vi "PTScanner.ProcCases.vi"(0 "i ref in":refnum<vi>, 1 "selector":string, 2 "Data":T3, 3 "call cluster":T1={"Object"="", "Selector"="", "CallType"=enum."synchronous", "Async Object"="", "Async Selector"="", "Data Descriptor"="", "Data"=[], "Error #"=0, "Expire"=0}, 5 "error in (no error)":errorcluster) -> (14 "i ref out":refnum<vi>, 17 "answer cluster":T1={"Object"="", "Selector"="", "CallType"=enum."synchronous", "Async Object"="", "Async Selector"="", "Data Descriptor"="", "Data"=[], "Error #"=0, "Expire"=0}, 19 "error out":errorcluster)   [LabVIEW 2014, in "PTScanner.lvlib"]
uses:
  PTScanner.lvlib
  CS_Core/CSSystem/CoreDefs/CoreDefs.rawDataType.ctl
  CS_Core/CSSystem/CoreDefs/CoreDefs.call_type.ctl
  CS_Core/BaseProcess/BaseProcess.descriptor string definition.ctl
  CS_Core/CSSystem/CoreLib/CoreLib.string 2 byte array.vi
  CS_Core/CSSystem/CoreLib/CoreLib.byte array 2 string.vi
  <vilib>/Utility/xml.llb/Write to XML File(string).vi
  <vilib>/Utility/xml.llb/Read From XML File(string).vi
  CS_Core/CSSystem/CoreLib/CoreLib.short 2 byte array.vi
  CS_Core/BaseProcess/BaseProcess.lvlib
  CS_Core/CSSystem/CoreLib/CoreLib.lvlib
  CS_Core/CAEObj/CAEObj.lvlib
  CSlibraries-extern/DimLVEvent/LVDimInterface/LVDimInterface.lvlib
  CS_Core/BaseSM/BaseSM.lvlib
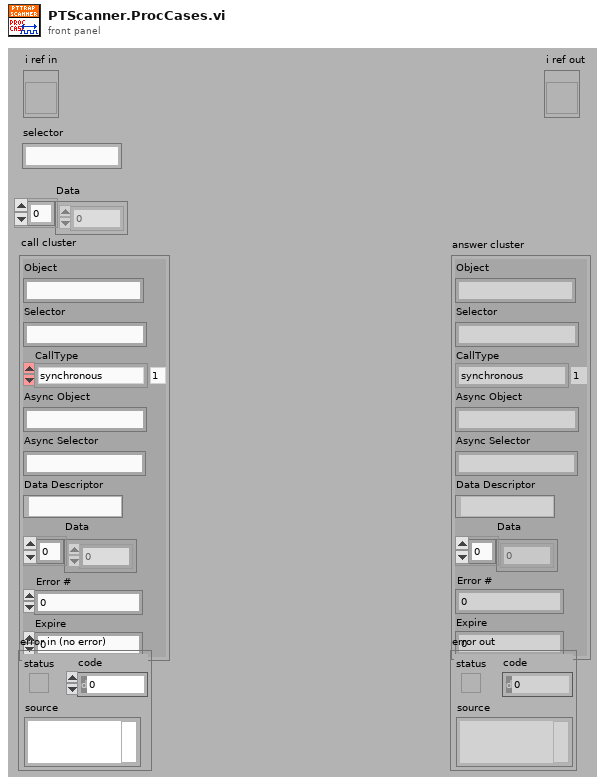
[diagram p1: front panel]
types:
  T1 = typedef "CoreDefs.call_type.ctl" = cluster{"Object":string, "Selector":string, "CallType":enum16{"simple", "synchronous", "asynchronous"}, "Async Object":string, "Async Selector":string, "Data Descriptor":T2, "Data":T3, "Error #":i32, "Expire":u32}
  T2 = typedef "BaseProcess.lvlib/BaseProcess.descriptor string definition.ctl" = string
  T3 = typedef "CoreDefs.rawDataType.ctl" = i8[]
  T4 = typedef "PTScanner.lvlib/PTScanner.i attribute.ctl" = cluster{"Object cmds":T5[], "Steps":cluster{"Finished":bool, "cmd setup":T6[]}[], "curStep":i32, "DIM IDs":cluster{"AllFinished":i32, "Finished":i32, "curStep":i32, "nofSteps":i32, "NomValues":i32[], "1D-Min":i32, "1D-Max":i32, "Dimensions":i32, "MaxDimensions":i32, "ScanedDeviceNames":i32[]}, "All Finished":bool, "DIMs in use":string[], "Running":bool, "Scan Delay":u32, "loop":bool, "Paused":bool, "Formed":bool}
  T5 = typedef "PTScanner.lvlib/PTScanner.obj parameters.ctl" = cluster{"object":string, "DIM address":string, "method":string, "data descriptor":string, "method parameters":cluster{"Name":string, "Descr":string, "Value":string, "Value?":bool}[], "Call Mode":enum16{"Simple DIM", "Synchronous"}, "actValue":dbl, "Centroid":dbl, "Minus Delta":dbl, "Plus Delta":dbl, "increment":dbl, "DIM Status":cluster{"no link":bool, "quality":i32, "Time Stamp":timestamp}, "range":dbl, "DIMChannelIndex":i32}
  T6 = typedef "PTScanner.lvlib/PTScanner.step obj parameters.ctl" = cluster{"obj index":i32, "nomValue":dbl, "fulfilled":bool}
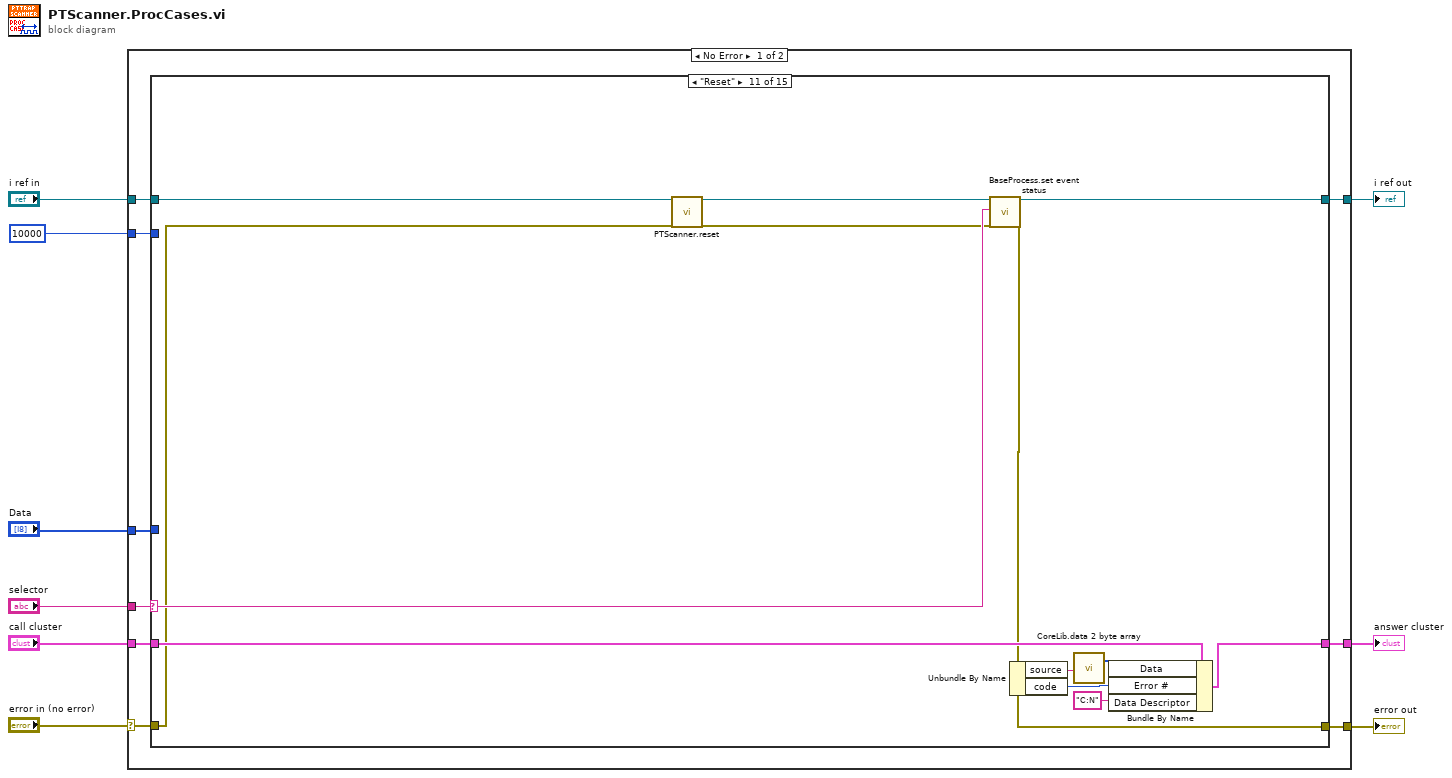
[diagram p0: block diagram]
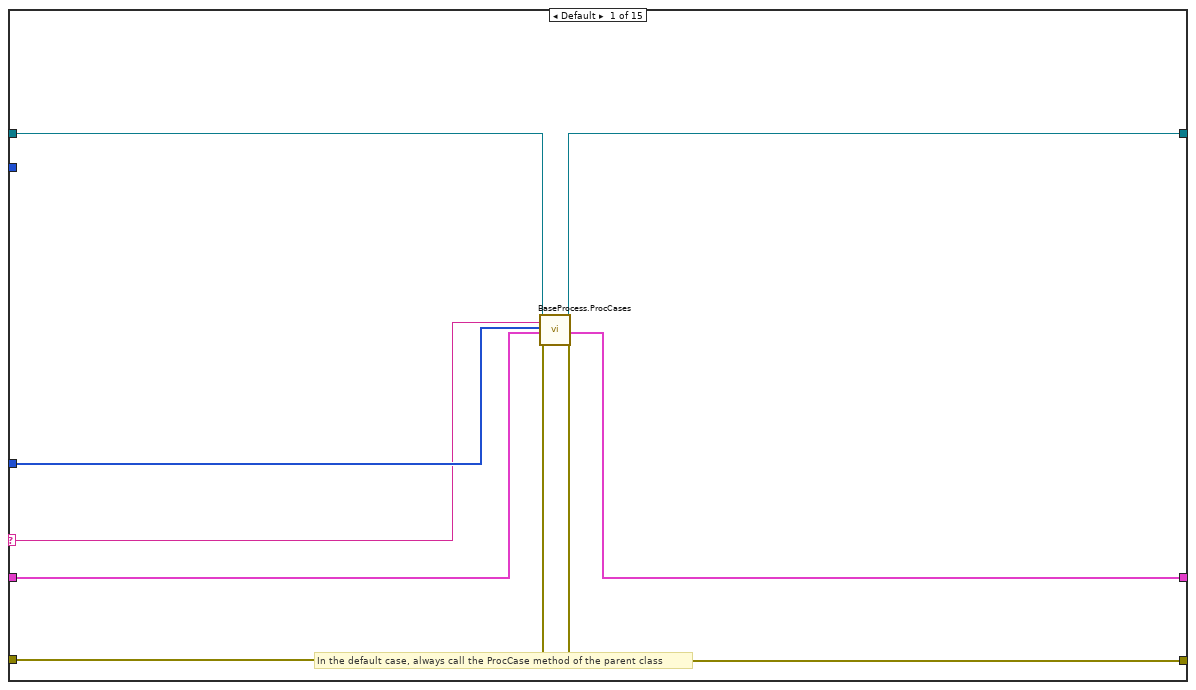
[diagram p2: hidden frame]
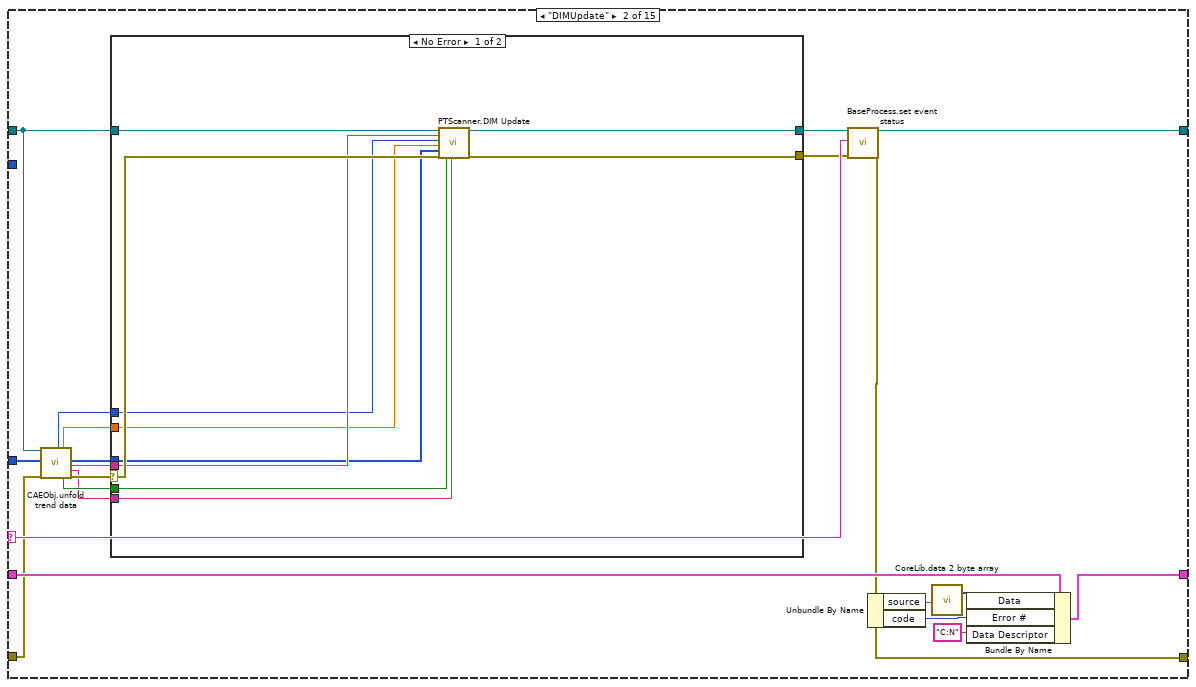
[diagram p3: hidden frame]
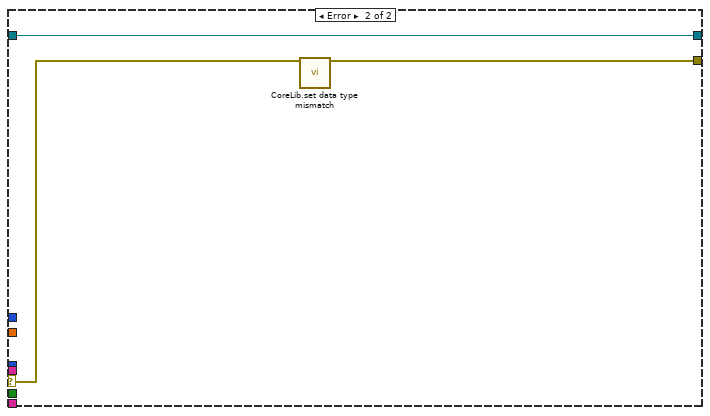
[diagram p4: hidden frame]
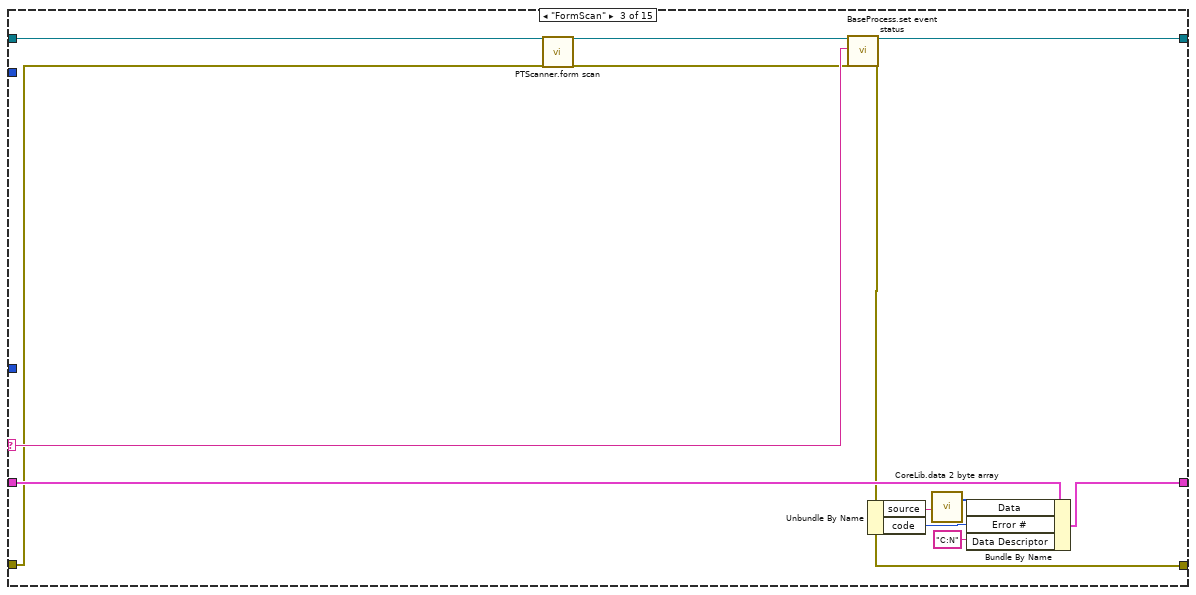
[diagram p5: hidden frame]
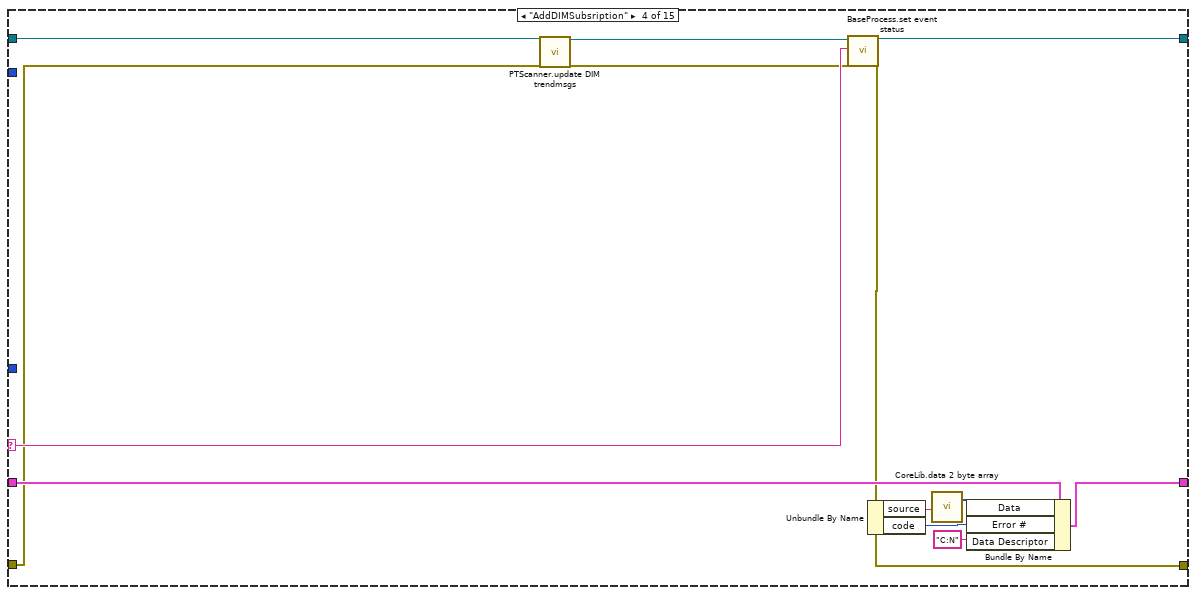
[diagram p6: hidden frame]
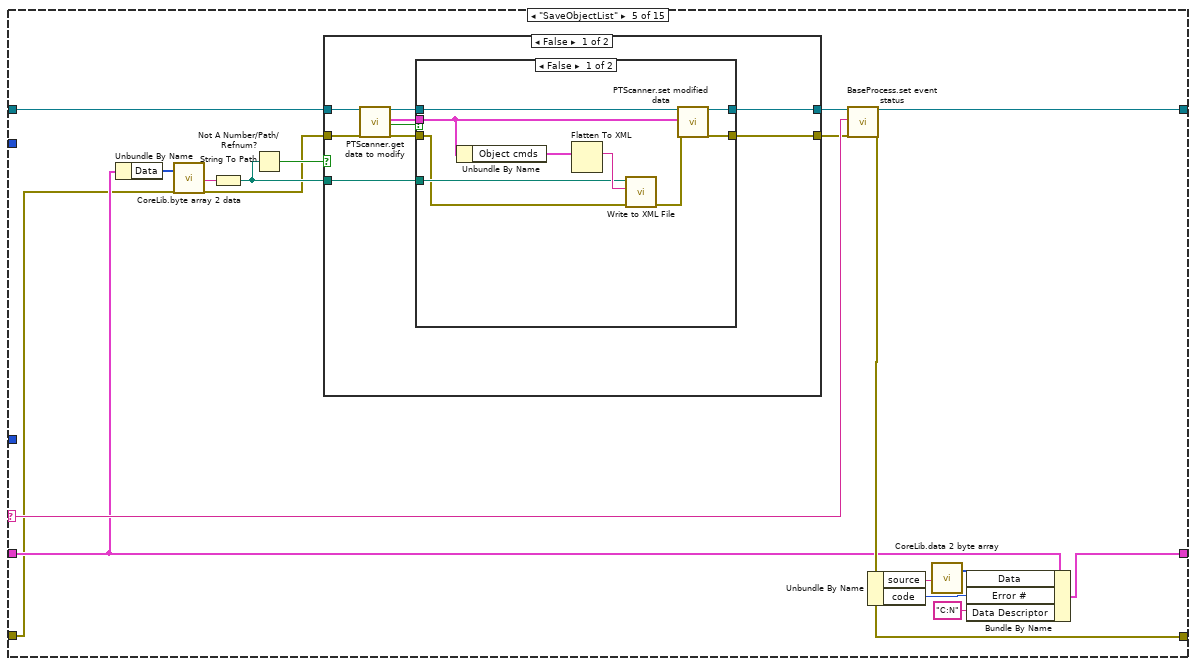
[diagram p7: hidden frame]
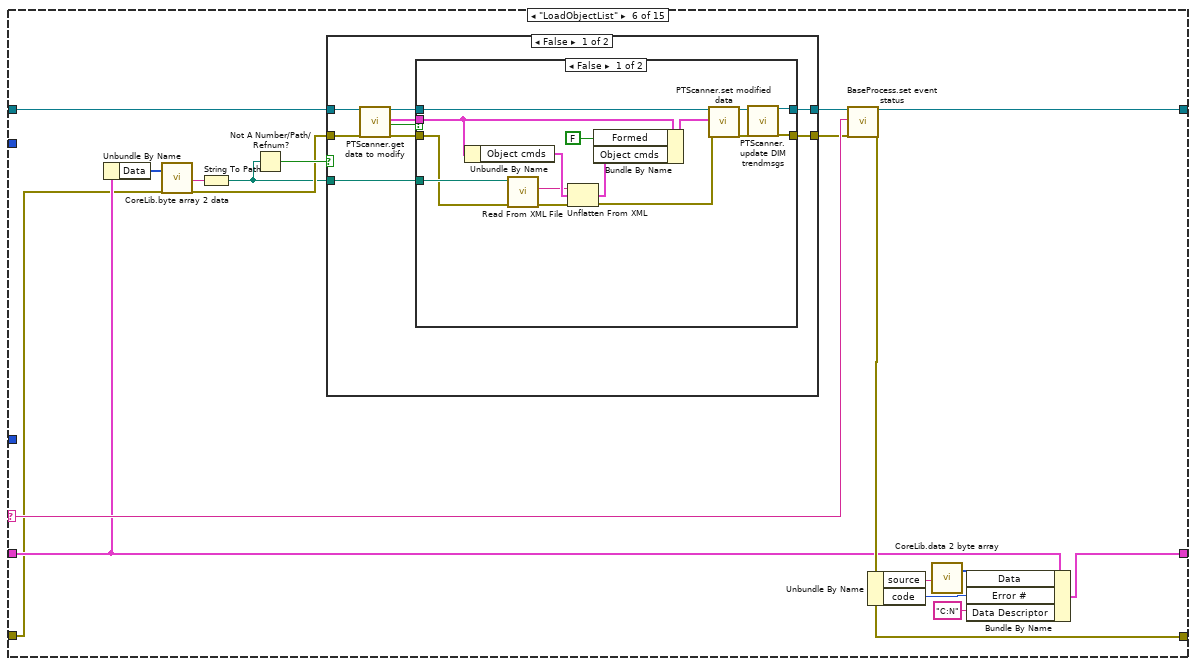
[diagram p10: hidden frame]
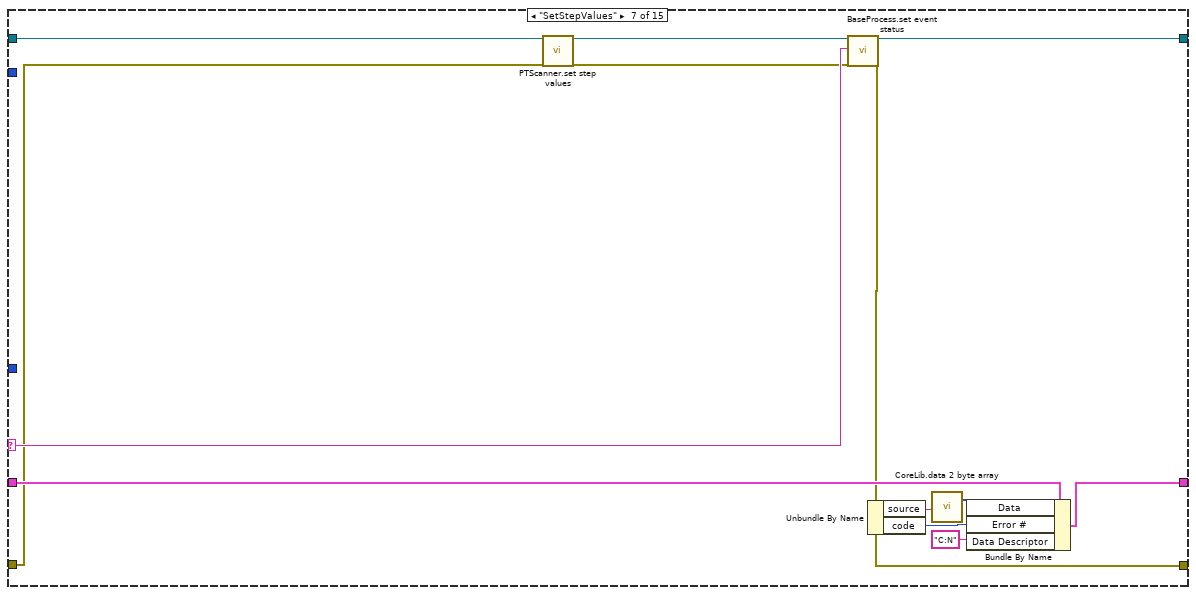
[diagram p13: hidden frame]
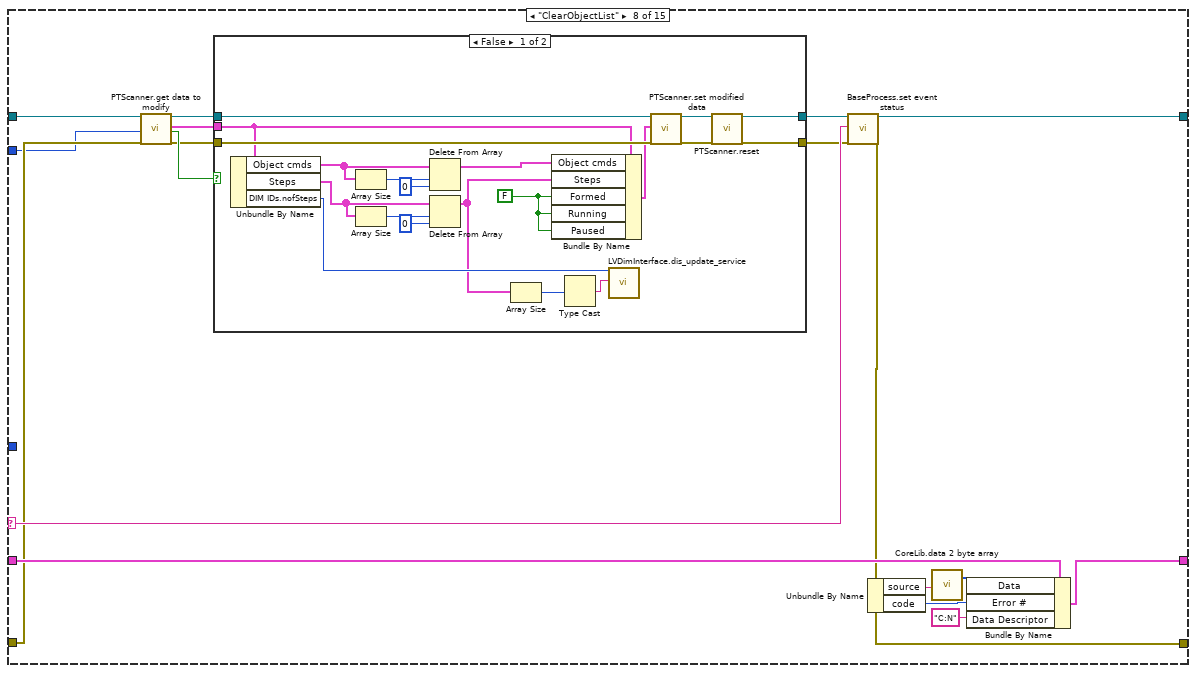
[diagram p14: hidden frame]
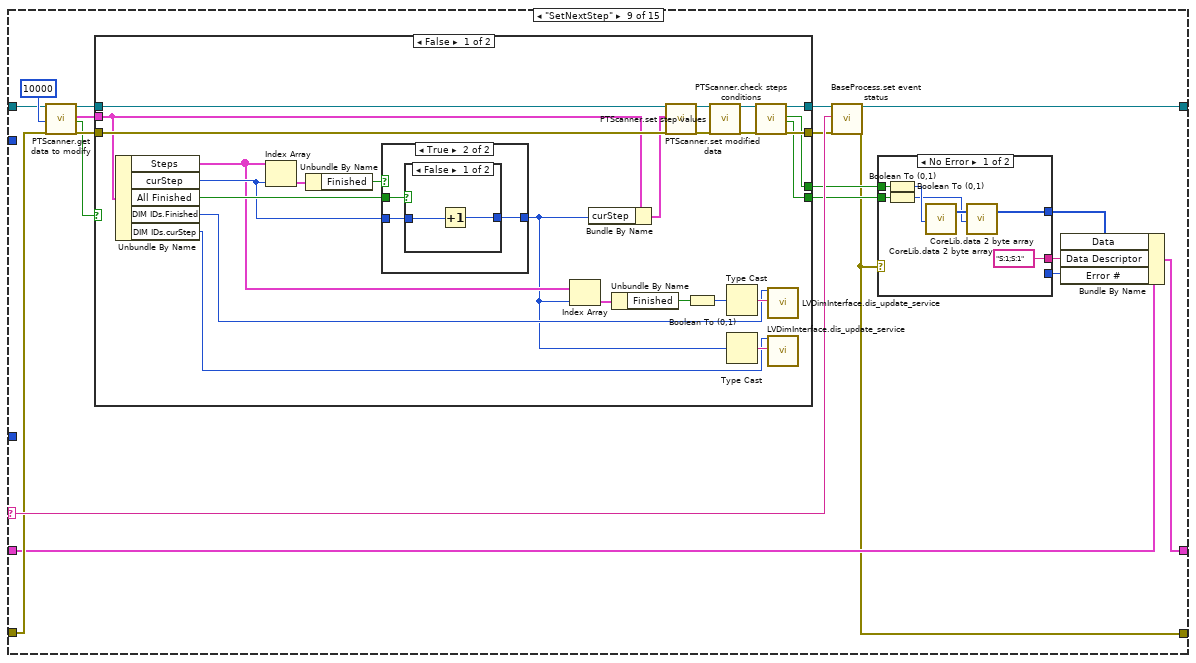
[diagram p16: hidden frame]
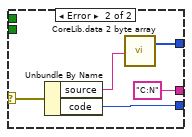
[diagram p17: hidden frame]
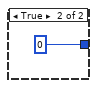
[diagram p19: hidden frame]
diagram:
  n1 = case shown="No Error" "error in (no error)" {
    selector: "error in (no error)" -> [w10 w504]
    tunnel: "selector" -> [w18 _]
    tunnel: [w17 w505] -> w8
    tunnel: "Data" -> [w16 _]
    tunnel: "call cluster" -> [w15 w505]
    tunnel: "i ref in" -> [w14 w506]
    tunnel: [w13 w506] -> w4
    tunnel: [w12 w504] -> w3
    tunnel: 10000 -> [w11 _]
    frame No Error {
      n2 = case shown="\"Reset\"" w18 {
        selector: w18 -> [w20 w39 w67 w80 w99 w139 w179 w197 w244 w306 w365 w378 w396 w451 w478]
        tunnel: w16 -> [w21 w38 _ _ _ _ _ _ _ _ _ _ _ _ _]
        tunnel: w14 -> [w19 w31 w65 w76 w88 w131 w177 w195 w235 w302 w362 w375 w392 w447 w474]
        tunnel: [w26 w41 w66 w79 w98 w138 w178 w196 w243 w305 w364 w377 w395 w450 w477] -> w13
        tunnel: w15 -> [w22 w43 w69 w82 w91 w134 w181 w199 w227 w307 w367 w380 w398 w453 w480]
        tunnel: [w23 w42 w70 w83 w101 w141 w182 w200 w228 w308 w368 w381 w399 w454 w481] -> w17
        tunnel: w10 -> [w25 w36 w64 w75 w90 w130 w174 w194 w234 w300 w361 w372 w390 w445 w472]
        tunnel: [w24 w40 w68 w81 w100 w140 w180 w198 w226 w295 w366 w379 w397 w452 w479] -> w12
        tunnel: w11 -> [_ _ _ _ _ _ _ w193 _ _ _ _ _ _ _]
        frame Default {
          # "In the default case, always call the ProcCase method of the parent class"
          n3 = call "BaseProcess.ProcCases.vi"("i ref in"=w19, "selector"=w20, "Data"=w21, "call cluster"=w22, "error in (no error)"=w25) -> ("i ref out"=w26:refnum<vi>, "answer cluster"=w23:T1, "error out"=w24:errorcluster)  [unwired: 12 in]
        }
        frame "DIMUpdate" {
          n4 = call "CAEObj.unfold trend data.vi"("i ref in"=w31, "raw trend data"=w38, "error in (no error)"=w36) -> ("quality"=w33:i32, "timeStamp"=w34:dbl, "no link"=w29:bool, "data"=w35:i8[], "serviceName"=w28:string, "typeDescriptor"=w27:string, "error out"=w37:errorcluster)  [unwired: 8 in, 2 out]
          n5 = case shown="No Error" w37 {
            selector: w37 -> [w54 w59]
            tunnel: w35 -> [w51 _]
            tunnel: w34 -> [w49 _]
            tunnel: w33 -> [w50 _]
            tunnel: [w55 w60] -> w32
            tunnel: w31 -> [w57 w58]
            tunnel: [w56 w58] -> w30
            tunnel: w29 -> [w53 _]
            tunnel: w28 -> [w52 _]
            tunnel: w27 -> [w48 _]
            frame No Error {
              n6 = call "PTScanner.DIM Update.vi"("i ref in"=w57, "serviceName"=w52, "quality"=w50, "Time Stamp"=w49, "data"=w51, "error in (no error)"=w54, "no link"=w53, "typeDescriptor"=w48) -> ("i ref out"=w56:refnum<vi>, "error out"=w55:errorcluster)  [unwired: 10 in]
            }
            frame Error {
              n7 = call "CoreLib.set data type mismatch.vi"("error in (no error)"=w59) -> ("error out"=w60:errorcluster)  [unwired: 18 in]
            }
          }
          n8 = call "BaseProcess.set event status.vi"("i ref in"=w30, "EventStatus"=w39, "error in (no error)"=w32) -> ("i ref out"=w41:refnum<vi>, "error out"=w40:errorcluster)  [unwired: 14 in, 1 out]
          n9 = Unbundle By Name(w40) -> ("source"=w44:string, "code"=w47:i32)
          n10 = call-poly "CoreLib.data 2 byte array.vi"("string"=w44) -> ("byteArray out"=w46:T3)  [unwired: 18 in]
          n11 = Bundle By Name(cluster=w43, "Data"=w46, "Error #"=w47, "Data Descriptor"="C:N") -> (w42:T1)
        }
        frame "FormScan" {
          n12 = call "PTScanner.form scan.vi"("i ref in"=w65, "error in (no error)"=w64) -> ("i ref out"=w63:refnum<vi>, "error out"=w62:errorcluster)  [unwired: 16 in]
          n13 = call "BaseProcess.set event status.vi"("i ref in"=w63, "EventStatus"=w67, "error in (no error)"=w62) -> ("i ref out"=w66:refnum<vi>, "error out"=w68:errorcluster)  [unwired: 14 in, 1 out]
          n14 = Unbundle By Name(w68) -> ("source"=w61:string, "code"=w73:i32)
          n15 = call-poly "CoreLib.data 2 byte array.vi"("string"=w61) -> ("byteArray out"=w72:T3)  [unwired: 18 in]
          n16 = Bundle By Name(cluster=w69, "Data"=w72, "Error #"=w73, "Data Descriptor"="C:N") -> (w70:T1)
        }
        frame "AddDIMSubsription" {
          n17 = call "PTScanner.update DIM trendmsgs.vi"("i ref in"=w76, "error in"=w75) -> ("i ref out"=w78:refnum<vi>, "error out"=w77:errorcluster)  [unwired: 16 in]
          n18 = call "BaseProcess.set event status.vi"("i ref in"=w78, "EventStatus"=w80, "error in (no error)"=w77) -> ("i ref out"=w79:refnum<vi>, "error out"=w81:errorcluster)  [unwired: 14 in, 1 out]
          n19 = Unbundle By Name(w81) -> ("source"=w74:string, "code"=w86:i32)
          n20 = call-poly "CoreLib.data 2 byte array.vi"("string"=w74) -> ("byteArray out"=w85:T3)  [unwired: 18 in]
          n21 = Bundle By Name(cluster=w82, "Data"=w85, "Error #"=w86, "Data Descriptor"="C:N") -> (w83:T1)
        }
        frame "SaveObjectList" {
          n22 = Unbundle By Name(w91) -> ("Data"=w95:T3)
          n23 = call-poly "CoreLib.byte array 2 data.vi"("byteArray"=w95, "error in (no error)"=w90) -> ("string"=w94:string, "error out"=w89:errorcluster)  [unwired: 15 in, 1 out]
          n24 = String To Path(string=w94) -> (path=w93:path)
          n25 = Not A Number/Path/Refnum?(number/path/refnum=w93) -> (NaN/Path/Refnum?=w92:bool)
          n26 = case shown="False" w92 {
            tunnel: w89 -> [w110 w125]
            tunnel: w88 -> [w113 w126]
            tunnel: w93 -> [w109 _]
            tunnel: [w107 w126] -> w97
            tunnel: [w105 w125] -> w96
            frame False {
              n27 = call "PTScanner.get data to modify.vi"("i ref in"=w113, "error in (no error)"=w110) -> ("i ref out"=w108:refnum<vi>, "i attribute"=w111:T4, "timed out"=w112:bool, "error out"=w106:errorcluster)  [unwired: 14 in]
              n28 = case shown="False" w112 {
                tunnel: w111 -> [w117 _]
                tunnel: w109 -> [w120 _]
                tunnel: [w119 w124] -> w107
                tunnel: w108 -> [w118 w124]
                tunnel: w106 -> [w116 w123]
                tunnel: [w114 w123] -> w105
                frame False {
                  n29 = Unbundle By Name(w117) -> ("Object cmds"=w122:T5[])
                  n30 = Flatten To XML(anything=w122) -> (xml string=w121:string)
                  n31 = call-poly <vilib>:"Write to XML File.vi"("error in (no error)"=w116, "XML Input"=w121, "XML File Path"=w120) -> ("error out"=w115:errorcluster)  [unwired: 6 in, 2 out]
                  n32 = call "PTScanner.set modified data.vi"("i ref in"=w118, "CLASS.i attribute"=w117, "error in (no error)"=w115) -> ("i ref out"=w119:refnum<vi>, "error out"=w114:errorcluster)  [unwired: 15 in]
                }
                frame True {
                }
              }
            }
            frame True {
            }
          }
          n33 = call "BaseProcess.set event status.vi"("i ref in"=w97, "EventStatus"=w99, "error in (no error)"=w96) -> ("i ref out"=w98:refnum<vi>, "error out"=w100:errorcluster)  [unwired: 14 in, 1 out]
          n34 = Unbundle By Name(w100) -> ("source"=w87:string, "code"=w104:i32)
          n35 = call-poly "CoreLib.data 2 byte array.vi"("string"=w87) -> ("byteArray out"=w103:T3)  [unwired: 18 in]
          n36 = Bundle By Name(cluster=w91, "Data"=w103, "Error #"=w104, "Data Descriptor"="C:N") -> (w101:T1)
        }
        frame "LoadObjectList" {
          n37 = Unbundle By Name(w134) -> ("Data"=w135:T3)
          n38 = call-poly "CoreLib.byte array 2 data.vi"("byteArray"=w135, "error in (no error)"=w130) -> ("string"=w133:string, "error out"=w129:errorcluster)  [unwired: 15 in, 1 out]
          n39 = String To Path(string=w133) -> (path=w128:path)
          n40 = Not A Number/Path/Refnum?(number/path/refnum=w128) -> (NaN/Path/Refnum?=w132:bool)
          n41 = case shown="False" w132 {
            tunnel: w129 -> [w150 w171]
            tunnel: w131 -> [w153 w172]
            tunnel: [w148 w172] -> w137
            tunnel: [w146 w171] -> w136
            tunnel: w128 -> [w145 _]
            frame False {
              n42 = call "PTScanner.get data to modify.vi"("i ref in"=w153, "error in (no error)"=w150) -> ("i ref out"=w149:refnum<vi>, "i attribute"=w151:T4, "timed out"=w152:bool, "error out"=w147:errorcluster)  [unwired: 14 in]
              n43 = case shown="False" w152 {
                tunnel: w151 -> [w163 _]
                tunnel: w145 -> [w168 _]
                tunnel: [w156 w170] -> w148
                tunnel: w149 -> [w167 w170]
                tunnel: w147 -> [w166 w169]
                tunnel: [w155 w169] -> w146
                frame False {
                  n44 = Unbundle By Name(w163) -> ("Object cmds"=w161:T5[])
                  n45 = call-poly <vilib>:"Read From XML File.vi"("error in (no error)"=w166, "XML File Path"=w168) -> ("error out"=w165:errorcluster, "XML Elements"=w160:string)  [unwired: 7 in, 1 out]
                  n46 = Unflatten From XML(xml string=w160, type=w161, error in (no error)=w165) -> (value=w162:T5[], error out=w164:errorcluster)
                  n47 = Bundle By Name(cluster=w163, "Formed"=FALSE, "Object cmds"=w162) -> (w159:T4)
                  n48 = call "PTScanner.set modified data.vi"("i ref in"=w167, "CLASS.i attribute"=w159, "error in (no error)"=w164) -> ("i ref out"=w158:refnum<vi>, "error out"=w157:errorcluster)  [unwired: 15 in]
                  n49 = call "PTScanner.update DIM trendmsgs.vi"("i ref in"=w158, "error in"=w157) -> ("i ref out"=w156:refnum<vi>, "error out"=w155:errorcluster)  [unwired: 16 in]
                }
                frame True {
                }
              }
            }
            frame True {
            }
          }
          n50 = call "BaseProcess.set event status.vi"("i ref in"=w137, "EventStatus"=w139, "error in (no error)"=w136) -> ("i ref out"=w138:refnum<vi>, "error out"=w140:errorcluster)  [unwired: 14 in, 1 out]
          n51 = Unbundle By Name(w140) -> ("source"=w127:string, "code"=w144:i32)
          n52 = call-poly "CoreLib.data 2 byte array.vi"("string"=w127) -> ("byteArray out"=w143:T3)  [unwired: 18 in]
          n53 = Bundle By Name(cluster=w134, "Data"=w143, "Error #"=w144, "Data Descriptor"="C:N") -> (w141:T1)
        }
        frame "SetStepValues" {
          n54 = call "PTScanner.set step values.vi"("i ref in"=w177, "error in(no error)"=w174) -> ("i ref out"=w176:refnum<vi>, "error out"=w175:errorcluster)  [unwired: 16 in]
          n55 = call "BaseProcess.set event status.vi"("i ref in"=w176, "EventStatus"=w179, "error in (no error)"=w175) -> ("i ref out"=w178:refnum<vi>, "error out"=w180:errorcluster)  [unwired: 14 in, 1 out]
          n56 = Unbundle By Name(w180) -> ("source"=w173:string, "code"=w185:i32)
          n57 = call-poly "CoreLib.data 2 byte array.vi"("string"=w173) -> ("byteArray out"=w184:T3)  [unwired: 18 in]
          n58 = Bundle By Name(cluster=w181, "Data"=w184, "Error #"=w185, "Data Descriptor"="C:N") -> (w182:T1)
        }
        frame "ClearObjectList" {
          n59 = call "PTScanner.get data to modify.vi"("i ref in"=w195, "ms timeout (10000)"=w193, "error in (no error)"=w194) -> ("i ref out"=w191:refnum<vi>, "i attribute"=w187:T4, "timed out"=w192:bool, "error out"=w190:errorcluster)  [unwired: 13 in]
          n60 = case shown="False" w192 {
            tunnel: w191 -> [w223 w225]
            tunnel: w190 -> [w222 w224]
            tunnel: [w210 w224] -> w189
            tunnel: [w209 w225] -> w188
            tunnel: w187 -> [w217 _]
            frame False {
              w208 = FALSE
              n61 = Unbundle By Name(w217) -> ("Object cmds"=w220:T5[], "Steps"=w213:cluster{"Finished":bool, "cmd setup":T6[]}[], "DIM IDs.nofSteps"=w206:i32)
              n62 = Array Size(array=w220) -> (size(s)=w221:i32)
              n63 = Array Size(array=w213) -> (size(s)=w214:i32)
              n64 = Delete From Array(array=w220, length=w221, index=0) -> (array with subset deleted=w218:T5[])  [unwired: 1 out]
              n65 = Delete From Array(array=w213, length=w214, index=0) -> (array with subset deleted=w205:cluster{"Finished":bool, "cmd setup":T6[]}[])  [unwired: 1 out]
              n66 = Array Size(array=w205) -> (size(s)=w204:i32)
              n67 = Bundle By Name(cluster=w217, "Object cmds"=w218, "Steps"=w205, "Formed"=w208, "Running"=w208, "Paused"=w208) -> (w216:T4)
              n68 = Type Cast(x=w204) -> (*(type *) &x=w207:string)  [unwired: 1 in]
              n69 = call "LVDimInterface.dis_update_service.vi"("my_serviceID"=w206, "data"=w207) -> ()  [unwired: 15 in, 3 out]
              n70 = call "PTScanner.set modified data.vi"("i ref in"=w223, "CLASS.i attribute"=w216, "error in (no error)"=w222) -> ("i ref out"=w212:refnum<vi>, "error out"=w211:errorcluster)  [unwired: 15 in]
              n71 = call "PTScanner.reset.vi"("i ref in"=w212, "error in (no error)"=w211) -> ("i ref out"=w209:refnum<vi>, "error out"=w210:errorcluster)  [unwired: 16 in]
            }
            frame True {
            }
          }
          n72 = call "BaseProcess.set event status.vi"("i ref in"=w188, "EventStatus"=w197, "error in (no error)"=w189) -> ("i ref out"=w196:refnum<vi>, "error out"=w198:errorcluster)  [unwired: 14 in, 1 out]
          n73 = Unbundle By Name(w198) -> ("source"=w186:string, "code"=w203:i32)
          n74 = call-poly "CoreLib.data 2 byte array.vi"("string"=w186) -> ("byteArray out"=w202:T3)  [unwired: 18 in]
          n75 = Bundle By Name(cluster=w199, "Data"=w202, "Error #"=w203, "Data Descriptor"="C:N") -> (w200:T1)
        }
        frame "SetNextStep" {
          n76 = call "PTScanner.get data to modify.vi"("i ref in"=w235, "ms timeout (10000)"=10000, "error in (no error)"=w234) -> ("i ref out"=w240:refnum<vi>, "i attribute"=w236:T4, "timed out"=w237:bool, "error out"=w239:errorcluster)  [unwired: 13 in]
          n77 = case shown="False" w237 {
            tunnel: w240 -> [w281 w290]
            tunnel: [w262 w290] -> w242
            tunnel: [w263 w289] -> w241
            tunnel: w239 -> [w280 w289]
            tunnel: w236 -> [w278 _]
            tunnel: [w261 _] -> w229
            tunnel: [w260 _] -> w230
            frame False {
              n78 = Unbundle By Name(w278) -> ("Steps"=w270:cluster{"Finished":bool, "cmd setup":T6[]}[], "curStep"=w274:i32, "All Finished"=w276:bool, "DIM IDs.Finished"=w267:i32, "DIM IDs.curStep"=w258:i32)
              n79 = Index Array(array=w270, index=w274) -> (element=w275:cluster{"Finished":bool, "cmd setup":T6[]})
              n80 = Unbundle By Name(w275) -> ("Finished"=w273:bool)
              n81 = case shown="True" w273 {
                tunnel: w276 -> [_ w285]
                tunnel: [w282 w284] -> w257
                tunnel: w274 -> [w282 w283]
                frame False {
                }
                frame True {
                  n82 = case shown="False" w285 {
                    tunnel: [w287 0] -> w284
                    tunnel: w283 -> [w286 _]
                    frame False {
                      n83 = Increment(x=w286) -> (x+1=w287:i32)
                    }
                    frame True {
                    }
                  }
                }
              }
              n84 = Index Array(array=w270, index=w257) -> (element=w269:cluster{"Finished":bool, "cmd setup":T6[]})
              n85 = Bundle By Name(cluster=w278, "curStep"=w257) -> (w277:T4)
              n86 = Unbundle By Name(w269) -> ("Finished"=w268:bool)
              n87 = call "PTScanner.set modified data.vi"("i ref in"=w281, "CLASS.i attribute"=w277, "error in (no error)"=w280) -> ("i ref out"=w266:refnum<vi>, "error out"=w279:errorcluster)  [unwired: 15 in]
              n88 = Boolean To (0,1)(Boolean=w268) -> (0, 1=w271:i16)
              n89 = call "PTScanner.set step values.vi"("i ref in"=w266, "error in(no error)"=w279) -> ("i ref out"=w265:refnum<vi>, "error out"=w264:errorcluster)  [unwired: 16 in]
              n90 = Type Cast(x=w271) -> (*(type *) &x=w272:string)  [unwired: 1 in]
              n91 = Type Cast(x=w257) -> (*(type *) &x=w259:string)  [unwired: 1 in]
              n92 = call "PTScanner.check steps conditions.vi"("i ref in"=w265, "error in (no error)"=w264) -> ("i ref out"=w262:refnum<vi>, "Finished"=w261:bool, "All Finished"=w260:bool, "error out"=w263:errorcluster)  [unwired: 14 in]
              n93 = call "LVDimInterface.dis_update_service.vi"("my_serviceID"=w267, "data"=w272) -> ()  [unwired: 15 in, 3 out]
              n94 = call "LVDimInterface.dis_update_service.vi"("my_serviceID"=w258, "data"=w259) -> ()  [unwired: 15 in, 3 out]
            }
            frame True {
            }
          }
          n95 = call "BaseProcess.set event status.vi"("i ref in"=w242, "EventStatus"=w244, "error in (no error)"=w241) -> ("i ref out"=w243:refnum<vi>, "error out"=w226:errorcluster)  [unwired: 14 in, 1 out]
          n96 = case shown="No Error" w226 {
            selector: w226 -> [_ w253]
            tunnel: [_ w256] -> w231
            tunnel: [w245 w255] -> w233
            tunnel: w229 -> [w250 _]
            tunnel: w230 -> [w249 _]
            tunnel: ["S:1;S:1" ("Data Descriptor") "C:N" ("Data Descriptor")] -> w232
            frame No Error {
              n97 = Boolean To (0,1)(Boolean=w250) -> (0, 1=w248:i16)
              n98 = Boolean To (0,1)(Boolean=w249) -> (0, 1=w247:i16)
              n99 = call-poly "CoreLib.data 2 byte array.vi"("i16"=w248) -> ("byteArray out"=w251:T3)  [unwired: 18 in]
              n100 = call-poly "CoreLib.data 2 byte array.vi"("byteArray"=w251, "i16"=w247) -> ("byteArray out"=w245:T3)  [unwired: 17 in]
            }
            frame Error {
              n101 = Unbundle By Name(w253) -> ("source"=w254:string, "code"=w256:i32)
              n102 = call-poly "CoreLib.data 2 byte array.vi"("string"=w254) -> ("byteArray out"=w255:T3)  [unwired: 18 in]
            }
          }
          n103 = Bundle By Name(cluster=w227, "Data"=w233, "Data Descriptor"=w232, "Error #"=w231) -> (w228:T1)
        }
        frame "SetPreviousStep" {
          n104 = call "PTScanner.get data to modify.vi"("i ref in"=w302, "ms timeout (10000)"=10000, "error in (no error)"=w300) -> ("i ref out"=w301:refnum<vi>, "i attribute"=w296:T4, "timed out"=w297:bool, "error out"=w299:errorcluster)  [unwired: 13 in]
          n105 = case shown="False" w297 {
            tunnel: w301 -> [w347 w358]
            tunnel: [w329 w358] -> w304
            tunnel: [w328 w357] -> w303
            tunnel: w299 -> [w346 w357]
            tunnel: w296 -> [w338 _]
            tunnel: [w327 _] -> w294
            tunnel: [w326 _] -> w293
            frame False {
              n106 = Unbundle By Name(w338) -> ("Steps"=w333:cluster{"Finished":bool, "cmd setup":T6[]}[], "curStep"=w341:i32, "DIM IDs.Finished"=w332:i32, "DIM IDs.curStep"=w324:i32)
              n107 = Array Size(array=w333) -> (size(s)=w340:i32)
              n108 = Index Array(array=w333, index=w341) -> (element=w344:cluster{"Finished":bool, "cmd setup":T6[]})
              n109 = Decrement(x=w340) -> (x-1=w339:i32)
              n110 = Equal To 0?(x=w341) -> (x = 0?=w342:bool)
              n111 = Unbundle By Name(w344) -> ("Finished"=w343:bool)
              n112 = case shown="True" w343 {
                tunnel: w342 -> [_ w353]
                tunnel: w341 -> [w349 w352]
                tunnel: w339 -> [_ w351]
                tunnel: [w349 w350] -> w322
                frame False {
                }
                frame True {
                  n113 = case shown="True" w353 {
                    tunnel: [w355 w356] -> w350
                    tunnel: w352 -> [w354 _]
                    tunnel: w351 -> [_ w356]
                    frame False {
                      n114 = Decrement(x=w354) -> (x-1=w355:i32)
                    }
                    frame True {
                    }
                  }
                }
              }
              n115 = Index Array(array=w333, index=w322) -> (element=w334:cluster{"Finished":bool, "cmd setup":T6[]})
              n116 = Bundle By Name(cluster=w338, "curStep"=w322) -> (w337:T4)
              n117 = Unbundle By Name(w334) -> ("Finished"=w323:bool)
              n118 = call "PTScanner.set modified data.vi"("i ref in"=w347, "CLASS.i attribute"=w337, "error in (no error)"=w346) -> ("i ref out"=w348:refnum<vi>, "error out"=w345:errorcluster)  [unwired: 15 in]
              n119 = Boolean To (0,1)(Boolean=w323) -> (0, 1=w335:i16)
              n120 = call "PTScanner.set step values.vi"("i ref in"=w348, "error in(no error)"=w345) -> ("i ref out"=w331:refnum<vi>, "error out"=w330:errorcluster)  [unwired: 16 in]
              n121 = Type Cast(x=w335) -> (*(type *) &x=w336:string)  [unwired: 1 in]
              n122 = Type Cast(x=w322) -> (*(type *) &x=w325:string)  [unwired: 1 in]
              n123 = call "PTScanner.check steps conditions.vi"("i ref in"=w331, "error in (no error)"=w330) -> ("i ref out"=w329:refnum<vi>, "Finished"=w327:bool, "All Finished"=w326:bool, "error out"=w328:errorcluster)  [unwired: 14 in]
              n124 = call "LVDimInterface.dis_update_service.vi"("my_serviceID"=w332, "data"=w336) -> ()  [unwired: 15 in, 3 out]
              n125 = call "LVDimInterface.dis_update_service.vi"("my_serviceID"=w324, "data"=w325) -> ()  [unwired: 15 in, 3 out]
            }
            frame True {
            }
          }
          n126 = call "BaseProcess.set event status.vi"("i ref in"=w304, "EventStatus"=w306, "error in (no error)"=w303) -> ("i ref out"=w305:refnum<vi>, "error out"=w295:errorcluster)  [unwired: 14 in, 1 out]
          n127 = case shown="No Error" w295 {
            selector: w295 -> [_ w318]
            tunnel: [_ w321] -> w291
            tunnel: [w310 w320] -> w309
            tunnel: w294 -> [w315 _]
            tunnel: w293 -> [w314 _]
            tunnel: ["S:1;S:1" ("Data Descriptor") "C:N" ("Data Descriptor")] -> w292
            frame No Error {
              n128 = Boolean To (0,1)(Boolean=w315) -> (0, 1=w313:i16)
              n129 = Boolean To (0,1)(Boolean=w314) -> (0, 1=w312:i16)
              n130 = call-poly "CoreLib.data 2 byte array.vi"("i16"=w313) -> ("byteArray out"=w316:T3)  [unwired: 18 in]
              n131 = call-poly "CoreLib.data 2 byte array.vi"("byteArray"=w316, "i16"=w312) -> ("byteArray out"=w310:T3)  [unwired: 17 in]
            }
            frame Error {
              n132 = Unbundle By Name(w318) -> ("source"=w319:string, "code"=w321:i32)
              n133 = call-poly "CoreLib.data 2 byte array.vi"("string"=w319) -> ("byteArray out"=w320:T3)  [unwired: 18 in]
            }
          }
          n134 = Bundle By Name(cluster=w307, "Data"=w309, "Data Descriptor"=w292, "Error #"=w291) -> (w308:T1)
        }
        frame "Reset" {
          n135 = call "PTScanner.reset.vi"("i ref in"=w362, "error in (no error)"=w361) -> ("i ref out"=w360:refnum<vi>, "error out"=w359:errorcluster)  [unwired: 16 in]
          n136 = call "BaseProcess.set event status.vi"("i ref in"=w360, "EventStatus"=w365, "error in (no error)"=w359) -> ("i ref out"=w364:refnum<vi>, "error out"=w366:errorcluster)  [unwired: 14 in, 1 out]
          n137 = Unbundle By Name(w366) -> ("source"=w363:string, "code"=w371:i32)
          n138 = call-poly "CoreLib.data 2 byte array.vi"("string"=w363) -> ("byteArray out"=w370:T3)  [unwired: 18 in]
          n139 = Bundle By Name(cluster=w367, "Data"=w370, "Error #"=w371, "Data Descriptor"="C:N") -> (w368:T1)
        }
        frame "SetCentralValues" {
          n140 = call "PTScanner.set central values.vi"("i ref in"=w375, "error in(no error)"=w372) -> ("i ref out"=w374:refnum<vi>, "error out"=w373:errorcluster)  [unwired: 16 in]
          n141 = call "BaseProcess.set event status.vi"("i ref in"=w374, "EventStatus"=w378, "error in (no error)"=w373) -> ("i ref out"=w377:refnum<vi>, "error out"=w379:errorcluster)  [unwired: 14 in, 1 out]
          n142 = Unbundle By Name(w379) -> ("source"=w376:string, "code"=w384:i32)
          n143 = call-poly "CoreLib.data 2 byte array.vi"("string"=w376) -> ("byteArray out"=w383:T3)  [unwired: 18 in]
          n144 = Bundle By Name(cluster=w380, "Data"=w383, "Error #"=w384, "Data Descriptor"="C:N") -> (w381:T1)
        }
        frame "Start" {
          n145 = call "PTScanner.get data to modify.vi"("i ref in"=w392, "ms timeout (10000)"=10000, "error in (no error)"=w390) -> ("i ref out"=w391:refnum<vi>, "i attribute"=w386:T4, "timed out"=w387:bool, "error out"=w389:errorcluster)  [unwired: 13 in]
          n146 = case shown="False" w387 {
            tunnel: w391 -> [w406 w439]
            tunnel: [w409 w439] -> w394
            tunnel: [w408 w438] -> w393
            tunnel: w389 -> [w405 w438]
            tunnel: w386 -> [w404 _]
            frame False {
              n147 = Unbundle By Name(w404) -> ("Formed"=w403:bool, "Paused"=w407:bool)
              n148 = case shown="True" w403 {
                tunnel: [w412 w420] -> w409
                tunnel: w406 -> [w413 w419]
                tunnel: w405 -> [w414 w418]
                tunnel: [w411 w417] -> w408
                tunnel: w407 -> [_ w416]
                tunnel: w404 -> [w410 w415]
                frame False {
                  n149 = call "PTScanner.set modified data.vi"("i ref in"=w413, "CLASS.i attribute"=w410, "error in (no error)"=w414) -> ("i ref out"=w412:refnum<vi>, "error out"=w411:errorcluster)  [unwired: 15 in]
                }
                frame True {
                  n150 = case shown="False" w416 {
                    tunnel: [w427 w435] -> w420
                    tunnel: w419 -> [w425 w437]
                    tunnel: w418 -> [w423 w436]
                    tunnel: [w426 w434] -> w417
                    tunnel: w415 -> [w421 w433]
                    frame False {
                      n151 = call "PTScanner.set modified data.vi"("i ref in"=w425, "CLASS.i attribute"=w421, "error in (no error)"=w423) -> ("i ref out"=w424:refnum<vi>, "error out"=w422:errorcluster)  [unwired: 15 in]
                      n152 = call "BaseSM.request state change.vi"("i ref in"=w424, "change"=TRUE, "error in (no error)"=w422, "requested state"="START", "allowed current states"=string[] ["S0", "IDLE"]) -> ("i ref out"=w427:refnum<vi>, "error out"=w426:errorcluster)  [unwired: 11 in, 2 out]
                    }
                    frame True {
                      n153 = Bundle By Name(cluster=w433, "Paused"=FALSE) -> (w432:T4)
                      n154 = call "PTScanner.set modified data.vi"("i ref in"=w437, "CLASS.i attribute"=w432, "error in (no error)"=w436) -> ("i ref out"=w435:refnum<vi>, "error out"=w434:errorcluster)  [unwired: 15 in]
                    }
                  }
                }
              }
            }
            frame True {
            }
          }
          n155 = call "BaseProcess.set event status.vi"("i ref in"=w394, "EventStatus"=w396, "error in (no error)"=w393) -> ("i ref out"=w395:refnum<vi>, "error out"=w397:errorcluster)  [unwired: 14 in, 1 out]
          n156 = Unbundle By Name(w397) -> ("source"=w385:string, "code"=w402:i32)
          n157 = call-poly "CoreLib.data 2 byte array.vi"("string"=w385) -> ("byteArray out"=w401:T3)  [unwired: 18 in]
          n158 = Bundle By Name(cluster=w398, "Data"=w401, "Error #"=w402, "Data Descriptor"="C:N") -> (w399:T1)
        }
        frame "Stop" {
          n159 = call "PTScanner.get data to modify.vi"("i ref in"=w447, "ms timeout (10000)"=10000, "error in (no error)"=w445) -> ("i ref out"=w446:refnum<vi>, "i attribute"=w441:T4, "timed out"=w442:bool, "error out"=w444:errorcluster)  [unwired: 13 in]
          n160 = case shown="False" w442 {
            tunnel: w446 -> [w464 w466]
            tunnel: [w462 w466] -> w449
            tunnel: [w461 w465] -> w448
            tunnel: w444 -> [w463 w465]
            tunnel: w441 -> [w460 _]
            frame False {
              w458 = FALSE
              n161 = Bundle By Name(cluster=w460, "Running"=w458, "Paused"=w458) -> (w459:T4)
              n162 = call "PTScanner.set modified data.vi"("i ref in"=w464, "CLASS.i attribute"=w459, "error in (no error)"=w463) -> ("i ref out"=w462:refnum<vi>, "error out"=w461:errorcluster)  [unwired: 15 in]
            }
            frame True {
            }
          }
          n163 = call "BaseProcess.set event status.vi"("i ref in"=w449, "EventStatus"=w451, "error in (no error)"=w448) -> ("i ref out"=w450:refnum<vi>, "error out"=w452:errorcluster)  [unwired: 14 in, 1 out]
          n164 = Unbundle By Name(w452) -> ("source"=w440:string, "code"=w457:i32)
          n165 = call-poly "CoreLib.data 2 byte array.vi"("string"=w440) -> ("byteArray out"=w456:T3)  [unwired: 18 in]
          n166 = Bundle By Name(cluster=w453, "Data"=w456, "Error #"=w457, "Data Descriptor"="C:N") -> (w454:T1)
        }
        frame "Pause" {
          n167 = call "PTScanner.get data to modify.vi"("i ref in"=w474, "ms timeout (10000)"=10000, "error in (no error)"=w472) -> ("i ref out"=w473:refnum<vi>, "i attribute"=w468:T4, "timed out"=w469:bool, "error out"=w471:errorcluster)  [unwired: 13 in]
          n168 = case shown="False" w469 {
            tunnel: w473 -> [w488 w503]
            tunnel: [w493 w503] -> w476
            tunnel: [w492 w502] -> w475
            tunnel: w471 -> [w487 w502]
            tunnel: w468 -> [w490 _]
            frame False {
              n169 = Unbundle By Name(w490) -> ("Running"=w489:bool)
              n170 = case shown="True" w489 {
                selector: w489 -> [_ w499]
                tunnel: [w495 w501] -> w491
                tunnel: w490 -> [w495 w500]
                tunnel: w488 -> [w496 w497]
                tunnel: w487 -> [w494 w498]
                tunnel: [w494 w498] -> w486
                tunnel: [w496 w497] -> w485
                frame False {
                }
                frame True {
                  n171 = Bundle By Name(cluster=w500, "Paused"=w499) -> (w501:T4)
                }
              }
              n172 = call "PTScanner.set modified data.vi"("i ref in"=w485, "CLASS.i attribute"=w491, "error in (no error)"=w486) -> ("i ref out"=w493:refnum<vi>, "error out"=w492:errorcluster)  [unwired: 15 in]
            }
            frame True {
            }
          }
          n173 = call "BaseProcess.set event status.vi"("i ref in"=w476, "EventStatus"=w478, "error in (no error)"=w475) -> ("i ref out"=w477:refnum<vi>, "error out"=w479:errorcluster)  [unwired: 14 in, 1 out]
          n174 = Unbundle By Name(w479) -> ("source"=w467:string, "code"=w484:i32)
          n175 = call-poly "CoreLib.data 2 byte array.vi"("string"=w467) -> ("byteArray out"=w483:T3)  [unwired: 18 in]
          n176 = Bundle By Name(cluster=w480, "Data"=w483, "Error #"=w484, "Data Descriptor"="C:N") -> (w481:T1)
        }
      }
    }
    frame Error {
    }
  }
  "answer cluster" <- w8
  "i ref out" <- w4
  "error out" <- w3
